vi "Calculate Event Durations.vi"(8 "error in":errorcluster, 10 "transitions":dbl[][](array[numeric]), 11 "waveform":waveform(dbl)={"t0"=timestamp(3473168073.631 s since 1904-01-01), "dt"=1e-08, "Y"=[], "attributes"=variant("Average Size"=variant(dbl 15.0), "Frequency (Hz)"=variant(dbl 1998.0127546741205), "MD5[0]"=variant(dbl 3432209604.0), "MD5[1]"=variant(dbl 1216260660.0), "MD5[2]"=variant(dbl 1007192998.0), "MD5[3]"=variant(dbl 1264973305.0), "NSamp"=variant(dbl 400000.0), "Number of Samples"=variant(dbl 400000.0), "Process Timestamp"=variant(dbl 3474981266.2031035), "Recvy Amp (V)"=variant(dbl 2.6382379145344714), "Recvy Amp (mA)"=variant(dbl 5.276475829068943), "Recvy Frequency (Hz)"=variant(dbl 1998.1571037522094), "Recvy Pulse Width (us)"=variant(dbl 12.432430276870729), "Recvy Trigger (s)"=variant(dbl 0.00044008000000000003), "Resistance (ohms)"=variant(dbl 500.0), "Samp Freq (MHz)"=variant(dbl 100.0), "Sample Frequency (MHz)"=variant(dbl 100.0), "Stim Amp (V)"=variant(dbl -2.3035646134631413), "Stim Amp (mA)"=variant(dbl -4.607129226926283), "Stim Frequency (Hz)"=variant(dbl 1997.8684055960314), "Stim Pulse Width (us)"=variant(dbl 12.07493911743164), "Stim Trigger (s)"=variant(dbl 0.00041221), "dt (us)"=variant(dbl 0.01))}) -> (0 "error out":errorcluster, 3 "waveform out":waveform(dbl)={"t0"=timestamp(3473175600.631 s since 1904-01-01), "dt"=nan, "Y"=[], "attributes"=variant("Average Size"=variant(dbl 15.0), "Frequency (Hz)"=variant(dbl nan), "Interphase Delay (us)"=variant(dbl nan), "MD5[0]"=variant(dbl 3432209604.0), "MD5[1]"=variant(dbl 1216260660.0), "MD5[2]"=variant(dbl 1007192998.0), "MD5[3]"=variant(dbl 1264973305.0), "NSamp"=variant(dbl 400000.0), "Number of Samples"=variant(dbl 400000.0), "Period Jitter (us rms)"=variant(dbl -0.0), "Process Timestamp"=variant(dbl 3474981266.2031035), "Recvy Amp (V)"=variant(dbl 2.6382379145344714), "Recvy Amp (mA)"=variant(dbl 5.276475829068943), "Recvy Frequency (Hz)"=variant(dbl 1998.1571037522094), "Recvy Pulse Width (us)"=variant(dbl nan), "Recvy Trigger (s)"=variant(dbl 0.00044008000000000003), "Resistance (ohms)"=variant(dbl 500.0), "Samp Freq (MHz)"=variant(dbl 100.0), "Sample Frequency (MHz)"=variant(dbl 100.0), "Stim Amp (V)"=variant(dbl -2.3035646134631413), "Stim Amp (mA)"=variant(dbl -4.607129226926283), "Stim Frequency (Hz)"=variant(dbl 1997.8684055960314), "Stim Pulse Width (us)"=variant(dbl nan), "Stim Trigger (s)"=variant(dbl 0.00041221), "dt (us)"=variant(dbl 0.01))})   [LabVIEW 2010]
doc: "This function calculates the Pulse Width (us), Frequency (Hz) . Period (us), and Duty Factor for the Stimulus portion of a bipolar pulse waveform. The results are stored as Waveform attributes in double precision floating point.\n\nPulse duration is measured between the points on the pulse equal to one-third of the pulse amplitude. (EN 45502-2-1:2003 Active Implant Medical Devices - Part 2-1, Measurement of implantable pulse generator and lead characteristics)\n\nNote: \"Pulse Width, full width at half maximum (FWHM), and half width at half maximum (HWHM) are, in general, deprecated terms because width is a word that denotes a spatial parameter whereas the parameter of interest is time.\" (Source: IEEE Standard 181-2003, Standard on Transitions, Pulses, and Related Waveforms)"
panel:
  out "Frequency (Hz)":dbl=nan format="%.3f"
  out "Period Jitter (us rms)":dbl=nan format="%.3f"
  out "Interphase Delay (us)":dbl=nan format="%.3f"
  out "Recvy Pulse Width (us)":dbl=nan format="%.3f"
  out "Stim Pulse Width (us)":dbl=nan format="%.3f"
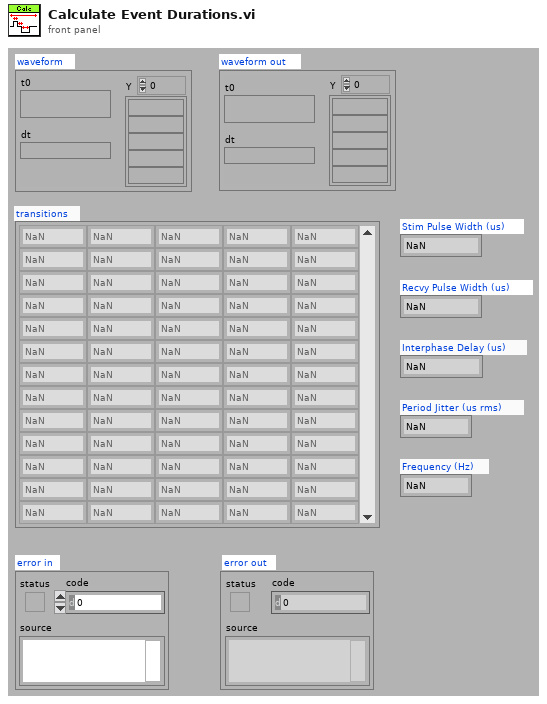
[diagram p1: front panel]
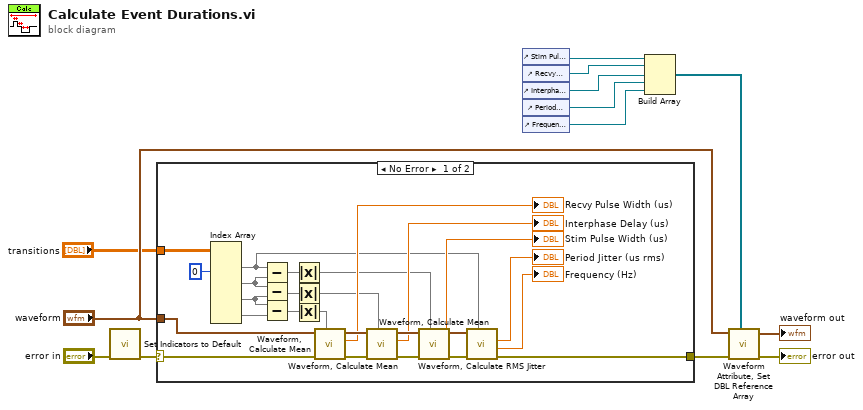
[diagram p0: block diagram]
diagram:
  n1 = call "Set Indicators to Default.vi"("error in"="error in") -> ("error out"=w7:errorcluster)  [unwired: 6 in]
  n2 = case shown="No Error" w7 {
    selector: w7 -> [w34 w40]
    tunnel: "waveform" -> [w28 _]
    tunnel: [w18 w40] -> w10
    tunnel: "transitions" -> [w39 _]
    frame No Error {
      n3 = Index Array(array=w39, index (col) #1=0 ("disabled index (col)")) -> (element #1=w17:dbl[], element #2=w35:dbl[], element #3=w36:dbl[], element #4=w37:dbl[])  [unwired: 7 in]
      n4 = Subtract(x=w17, y=w35) -> (x-y=w31:dbl[])
      n5 = Subtract(x=w35, y=w36) -> (x-y=w23:dbl[])
      n6 = Subtract(x=w36, y=w37) -> (x-y=w22:dbl[])
      n7 = Absolute Value(x=w31) -> (abs(x)=w24:dbl[])
      n8 = Absolute Value(x=w23) -> (abs(x)=w21:dbl[])
      n9 = Absolute Value(x=w22) -> (abs(x)=w20:dbl[])
      n10 = call "Waveform, Calculate Mean.vi"("error in"=w34, "waveform"=w28, "index"=w20) -> ("error out"=w33:errorcluster, "mean (us)"=→"Recvy Pulse Width (us)":dbl, "waveform dup"=w29:waveform(dbl))  [unwired: 5 in]
      n11 = call "Waveform, Calculate Mean.vi"("error in"=w33, "waveform"=w29, "index"=w21) -> ("error out"=w32:errorcluster, "mean (us)"=→"Interphase Delay (us)":dbl, "waveform dup"=w30:waveform(dbl))  [unwired: 5 in]
      n12 = call "Waveform, Calculate Mean.vi"("error in"=w32, "waveform"=w30, "index"=w24) -> ("error out"=w19:errorcluster, "mean (us)"=→"Stim Pulse Width (us)":dbl, "waveform dup"=w14:waveform(dbl))  [unwired: 5 in]
      n13 = call "Waveform, Calculate RMS Jitter.vi"("error in"=w19, "waveform"=w14, "transition index"=w17) -> ("error out"=w18:errorcluster, "Frequency (Hz)"=→"Frequency (Hz)":dbl, "Period Jitter (us rms)"=→"Period Jitter (us rms)":dbl)  [unwired: 4 in, 1 out]
    }
    frame Error {
    }
  }
  n14 = control-ref of="Stim Pulse Width (us)"() -> (w5:refnum<vi>)
  n15 = control-ref of="Recvy Pulse Width (us)"() -> (w4:refnum<vi>)
  n16 = control-ref of="Interphase Delay (us)"() -> (w3:refnum<vi>)
  n17 = control-ref of="Period Jitter (us rms)"() -> (w2:refnum<vi>)
  n18 = control-ref of="Frequency (Hz)"() -> (w1:refnum<vi>)
  n19 = Build Array(w5, w4, w3, w2, w1) -> (w13:refnum<vi>[])
  n20 = call "Waveform Attribute, Set DBL Reference Array.vi"("Refnum Array"=w13, "error in"=w10, "waveform"="waveform") -> ("error out"=→"error out":errorcluster, "waveform out"=→"waveform out":waveform(dbl))  [unwired: 5 in]
